vi "App Name.vi"(11 "DemoApp in":refnum<class "DemoApp.lvclass">) -> (2 "App Name":string)   [LabVIEW 2020, in "VolatusDemo.lvlib" / "DemoApp.lvclass"]
uses:
  DemoApp.lvclass
  DemoApp.lvclass/DemoApp.ctl
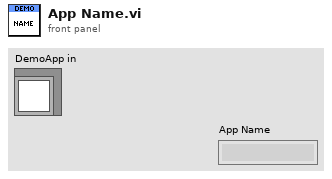
[diagram p1: front panel]
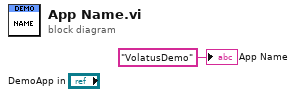
[diagram p0: block diagram]
diagram:
  "App Name" <- "VolatusDemo" ("App Name")
